vi "Convert ROI.vi"(1 "ROI":T1) -> (0 "Camera ROI":T2)   [LabVIEW 2020]
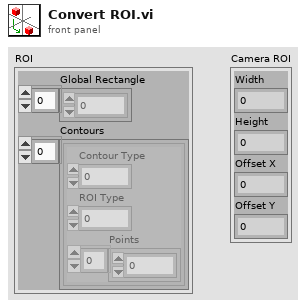
[diagram p1: front panel]
types:
  T1 = cluster{"Global Rectangle":i32[], "Contours":cluster{"Contour Type":u32, "ROI Type":u32, "Points":i32[]}[]}
  T2 = cluster{"Width":u32, "Height":u32, "Offset X":u32, "Offset Y":u32}
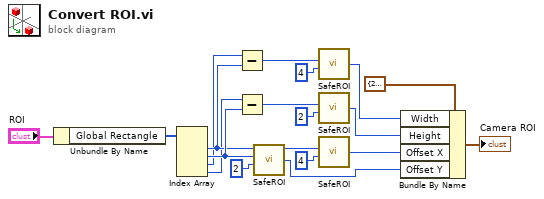
[diagram p0: block diagram]
diagram:
  n1 = Unbundle By Name("ROI") -> ("Global Rectangle"=w3:i32[])
  n2 = Index Array(array=w3) -> (element #1=w11:i32, element #2=w17:i32, element #3=w5:i32, element #4=w4:i32)  [unwired: 4 in]
  n3 = Subtract(x=w5, y=w11) -> (x-y=w8:i32)
  n4 = Subtract(x=w4, y=w17) -> (x-y=w13:i32)
  n5 = call "SafeROI.vi"("ROI in"=w17, "Increament"=2 ("2")) -> ("Safe ROI"=w18:u32)  [unwired: 6 in]
  n6 = call "SafeROI.vi"("ROI in"=w8, "Increament"=4 ("4")) -> ("Safe ROI"=w9:u32)  [unwired: 6 in]
  n7 = call "SafeROI.vi"("ROI in"=w13, "Increament"=2 ("2")) -> ("Safe ROI"=w14:u32)  [unwired: 6 in]
  n8 = call "SafeROI.vi"("ROI in"=w11, "Increament"=4 ("4")) -> ("Safe ROI"=w12:u32)  [unwired: 6 in]
  n9 = Bundle By Name(cluster=T2 {"Width"=2048, "Height"=2048, "Offset X"=0, "Offset Y"=0} ("Camera ROI"), "Width"=w9, "Height"=w14, "Offset X"=w12, "Offset Y"=w18) -> (→"Camera ROI":T2)
